vi "S2C_FORNAX_Proc_ShowMenu.vi"(8 "Error In":errorcluster, 9 "Cell Position":T1, 10 "MenuRef":refnum<k9>, 11 "CtlRef":refnum<vi>) -> (0 "Error Out":errorcluster, 3 "Discard?":bool)   [LabVIEW 2015]
doc: "Loads the popup menu for the selected Fornax command parameter."
uses:
  <vilib>/Utility/miscctls.llb/LVRowAndColumnTypeDef.ctl
  S2C_FORNAX_Proc_Globals.vi
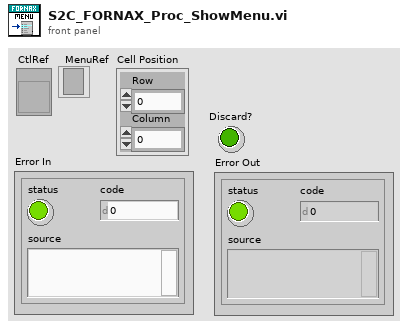
[diagram p1: front panel]
types:
  T1 = typedef "LVRowAndColumnTypeDef.ctl" = cluster{"Row":i32, "Column":i32}
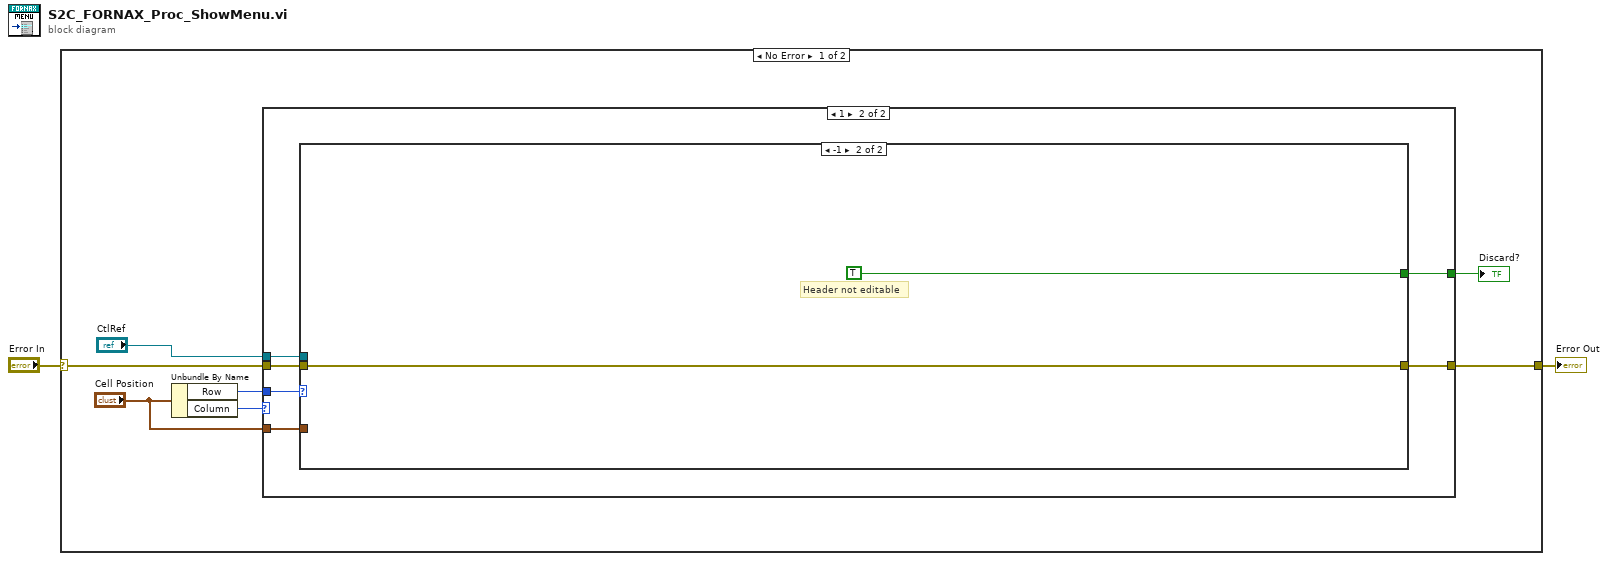
[diagram p0: block diagram]
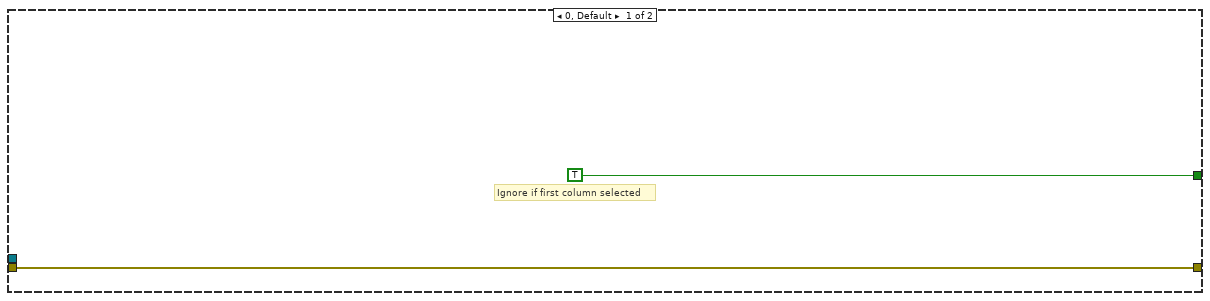
[diagram p2: hidden frame]
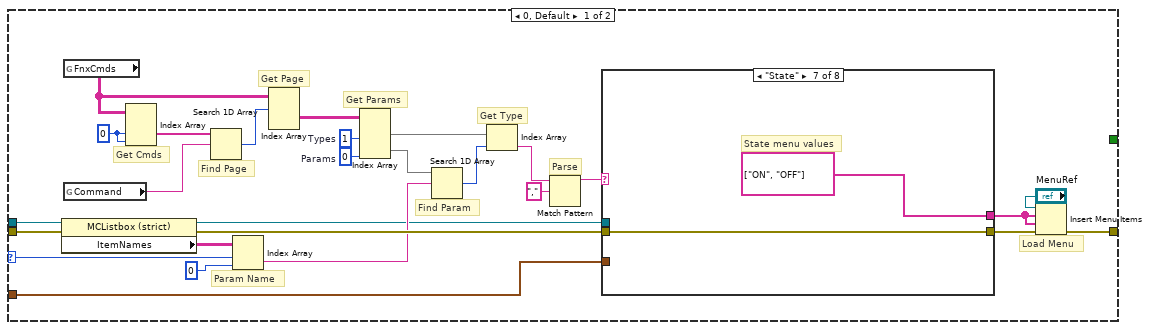
[diagram p3: hidden frame]
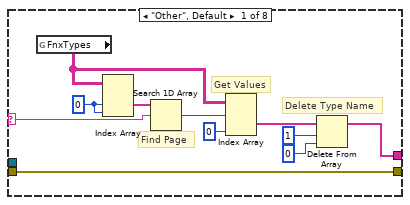
[diagram p4: hidden frame]
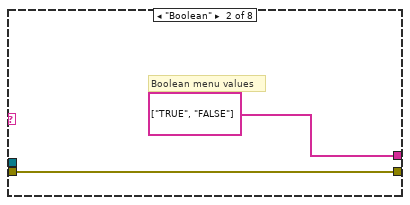
[diagram p5: hidden frame]
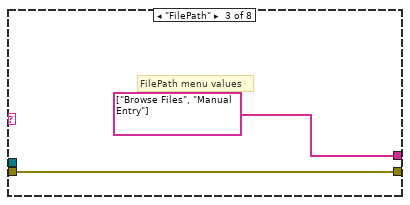
[diagram p6: hidden frame]
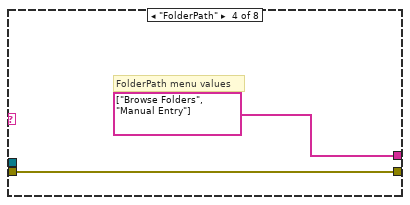
[diagram p7: hidden frame]
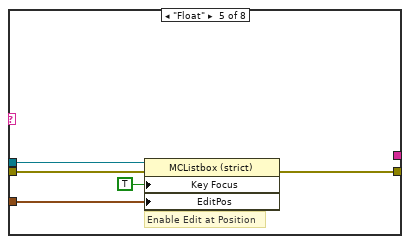
[diagram p8: hidden frame]
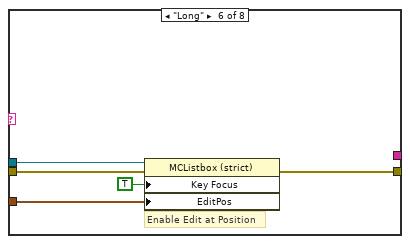
[diagram p9: hidden frame]
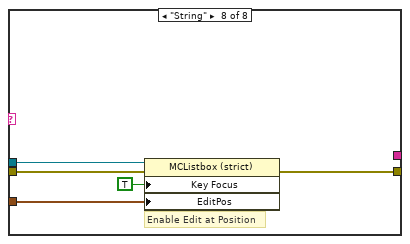
[diagram p10: hidden frame]
diagram:
  n1 = case shown="No Error" "Error In" {
    selector: "Error In" -> [w9 w80]
    tunnel: [w8 w80] -> w1
    frame No Error {
      n2 = Unbundle By Name("Cell Position") -> ("Row"=w7:i32, "Column"=w4:i32)
      n3 = case shown="1" w4 {
        tunnel: w9 -> [w11 w17]
        tunnel: [w11 w16] -> w8
        tunnel: w7 -> [_ w15]
        tunnel: [TRUE w14] -> w6
        tunnel: "Cell Position" -> [_ w13]
        tunnel: "CtlRef" -> [_ w12]
        frame 0, Default {
          # "Ignore if first column selected"
        }
        frame 1 {
          n4 = case shown="-1" w15 {
            selector: w15 -> [w38 _]
            tunnel: w17 -> [w40 w79]
            tunnel: [w39 w79] -> w16
            tunnel: [_ TRUE] -> w14
            tunnel: w13 -> [w24 _]
            tunnel: w12 -> [w23 _]
            frame 0, Default {
              w32 = 0  # Params
              w33 = 1  # Types
              w36 = 0 ("disabled index (row)")
              # "Parse"
              # "Load Menu"
              # "Get Type"
              # "Find Param"
              # "Get Params"
              # "Get Page"
              # "Find Page"
              # "Get Cmds"
              # "Param Name"
              n5 = property on="Property Node" class="MCListbox (strict)"(reference=w23, error in=w40) -> (reference out=w25:refnum<vi>, error out=w41:errorcluster, "ItemNames"=w43:string[][])
              n6 = global read "S2C_FORNAX_Proc_Globals.vi" "FnxCmds"() -> (w19:string[][][])
              n7 = global read "S2C_FORNAX_Proc_Globals.vi" "Command"() -> (w18:string)
              n8 = Index Array(array=w19, index (dim 1)=w36, index (dim 2)=w36) -> (element=w37:string[])  [unwired: 1 in]
              n9 = Search 1D Array(1D array=w37, element=w18) -> (index of element=w35:i32)  [unwired: 1 in]
              n10 = Index Array(array=w43, index (row)=w38, index (col)=0 ("disabled index (col)")) -> (element=w28:string)
              n11 = Index Array(array=w19, index (dim 0)=w35) -> (element=w34:string[][])  [unwired: 2 in]
              n12 = Index Array(array=w34, index (col) #1=w33, index (col) #2=w32) -> (element #1=w30:string[], element #2=w31:string[])  [unwired: 2 in]
              n13 = Search 1D Array(1D array=w31, element=w28) -> (index of element=w29:i32)  [unwired: 1 in]
              n14 = Index Array(array=w30, index=w29) -> (element=w22:string)
              n15 = Match Pattern(string=w22, regular expression=",") -> (before substring=w20:string)  [unwired: 1 in, 3 out]
              n16 = case shown="\"State\"" w20 {
                selector: w20 -> [w47 _ _ _ _ _ _ _]
                tunnel: w41 -> [w46 w56 w58 w60 w64 w69 w72 w76]
                tunnel: [w46 w56 w58 w60 w63 w68 w72 w75] -> w39
                tunnel: [w45 string[] ["TRUE", "FALSE"] string[] ["Browse Files", "Manual Entry"] string[] ["Browse Folders", "Manual Entry"] _ _ string[] ["ON", "OFF"] _] -> w26
                tunnel: w25 -> [_ _ _ _ w62 w67 _ w74]
                tunnel: w24 -> [_ _ _ _ w61 w66 _ w73]
                frame "Other", Default {
                  w54 = 0 ("disabled index (row)")
                  # "Delete Type Name"
                  # "Get Values"
                  # "Find Page"
                  n17 = global read "S2C_FORNAX_Proc_Globals.vi" "FnxTypes"() -> (w44:string[][][])
                  n18 = Index Array(array=w44, index (dim 1)=w54, index (dim 2)=w54) -> (element=w53:string[])  [unwired: 1 in]
                  n19 = Search 1D Array(1D array=w53, element=w47) -> (index of element=w52:i32)  [unwired: 1 in]
                  n20 = Index Array(array=w44, index (dim 0)=w52, index (dim 2)=0 ("disabled index (col)")) -> (element=w50:string[])  [unwired: 1 in]
                  n21 = Delete From Array(array=w50, length=1, index=0) -> (array with subset deleted=w45:string[])  [unwired: 1 out]
                }
                frame "Boolean" {
                  # "Boolean menu values"
                }
                frame "FilePath" {
                  # "FilePath menu values"
                }
                frame "FolderPath" {
                  # "FolderPath menu values"
                }
                frame "Float" {
                  # "Enable Edit at Position"
                  n22 = property on="Property Node" class="MCListbox (strict)"(reference=w62, error in=w64, "Key Focus"=TRUE, "EditPos"=w61) -> (error out=w63:errorcluster)  [unwired: 1 out]
                }
                frame "Long" {
                  # "Enable Edit at Position"
                  n23 = property on="Property Node" class="MCListbox (strict)"(reference=w67, error in=w69, "Key Focus"=TRUE, "EditPos"=w66) -> (error out=w68:errorcluster)  [unwired: 1 out]
                }
                frame "State" {
                  # "State menu values"
                }
                frame "String" {
                  # "Enable Edit at Position"
                  n24 = property on="Property Node" class="MCListbox (strict)"(reference=w74, error in=w76, "Key Focus"=TRUE, "EditPos"=w73) -> (error out=w75:errorcluster)  [unwired: 1 out]
                }
              }
              n25 = Insert Menu Items(7:w26, 8:w26, 9:"MenuRef") -> ()  [unwired: 3 in, 3 out]
            }
            frame -1 {
              # "Header not editable"
            }
          }
        }
      }
      "Discard?" <- w6
    }
    frame Error {
    }
  }
  "Error Out" <- w1
